vi "PreviousMonth.vi"(8 "error in (no error)":errorcluster, 11 "Calendar in":refnum<class "Calendar.lvclass">) -> (0 "error out":errorcluster, 3 "Calendar (dup)":refnum<class "Calendar.lvclass">)   [LabVIEW 2015, in "Calendar.lvclass"]
uses:
  Calendar.lvclass
  Calendar.lvclass/Calendar.ctl
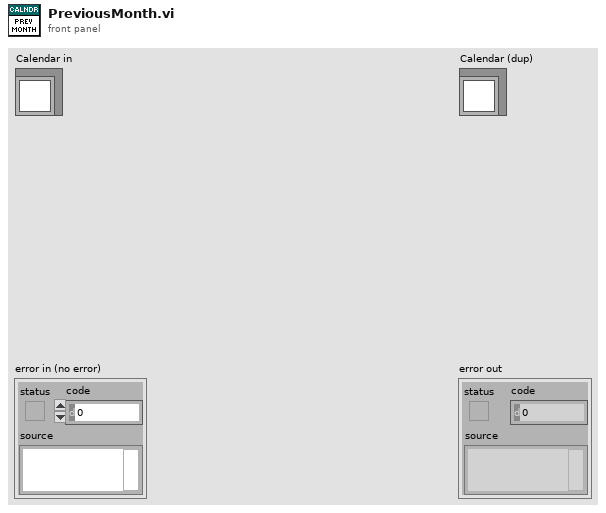
[diagram p1: front panel]
types:
  T1 = typedef "Calendar.lvclass/State Data.ctl" = cluster{"Current Date":timestamp, "First Day of Week":T2, "Color":cluster{"Selector Background":u32, "Selector Text":u32, "Days of Week Background":u32, "Days of Week Text":u32, "Calendar Background":u32, "Calendar Text":u32, "Calendar Selection Background":u32, "Calendar Selection Text":u32}, "Visible":cluster{"Today Selector Visible":bool, "Month-Year Selector Visible":bool}}
  T2 = typedef "Calendar.lvclass/DaysOfWeek.ctl" = enum16{"Sunday", "Monday", "Tuesday", "Wednesday", "Thursday", "Friday", "Saturday"}
  T3 = typedef "LVDateTimeRec.ctl" = cluster{"fractional second":dbl, "second":i32, "minute":i32, "hour":i32, "day of month":i32, "month":i32, "year":i32, "day of week":i32, "day of year":i32, "DST":i32}
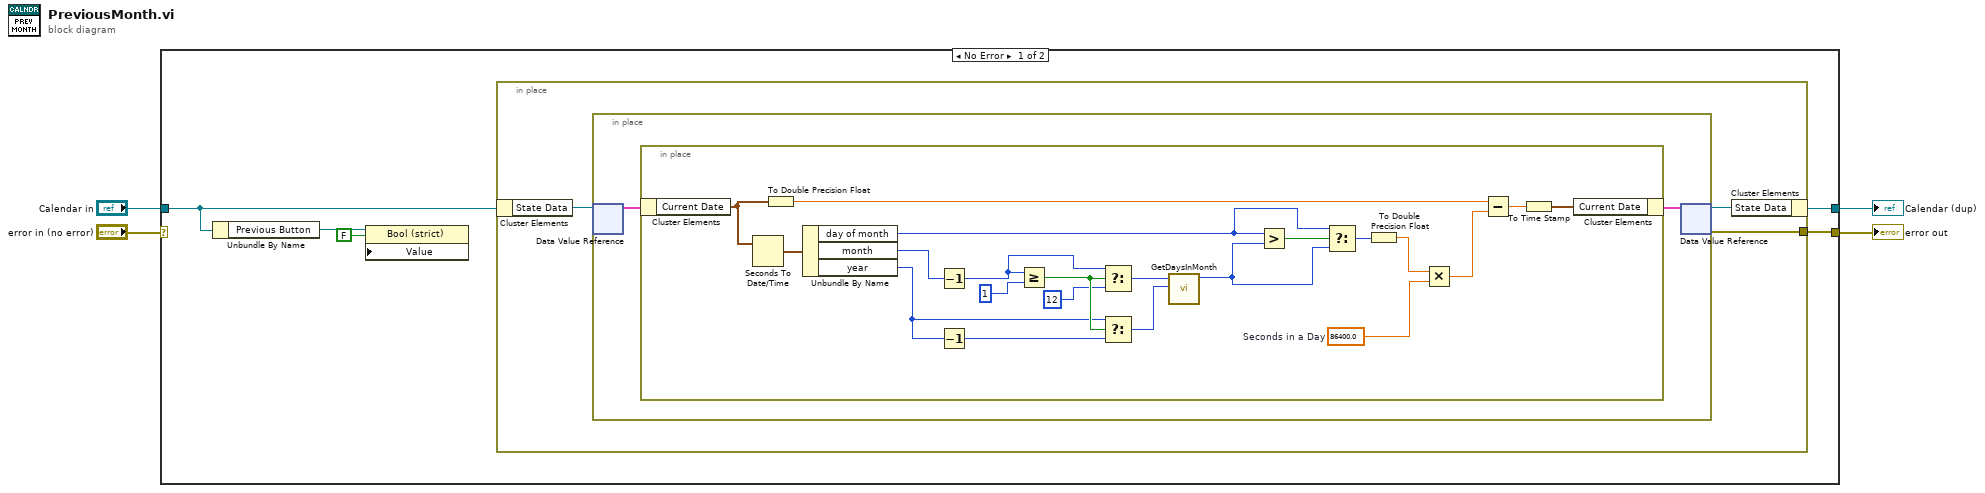
[diagram p0: block diagram]
diagram:
  n1 = case shown="No Error" "error in (no error)" {
    selector: "error in (no error)" -> [_ w37]
    tunnel: [w8 w37] -> w3
    tunnel: [w9 w36] -> w1
    tunnel: "Calendar in" -> [w7 w36]
    frame No Error {
      n2 = Unbundle By Name(w7) -> ("Previous Button"=w6:refnum<vi>)
      n3 = property class="Bool (strict)"(reference=w6, "Value"=FALSE) -> ()  [unwired: 1 in, 2 out]
      n4 = in-place {
        in-place-border: [w10] -> w8
        n5 = in-place-cluster #1(w7) -> ("State Data"=w12:refnum<data-value>)
        n6 = in-place {
          n7 = in-place-dvr #2(w12) -> (w14:T1)  [unwired: 1 out]
          n8 = in-place {
            w18 = 86400.0  # Seconds in a Day
            n9 = in-place-cluster #3(w14) -> ("Current Date"=w28:timestamp)
            n10 = Seconds To Date/Time(time stamp (now)=w28) -> (date time rec=w35:T3)  [unwired: 1 in]
            n11 = To Double Precision Float(number=w28) -> (double precision float=w27:dbl)
            n12 = Unbundle By Name(w35) -> ("day of month"=w15:i32, "month"=w24:i32, "year"=w22:i32)
            n13 = Decrement(x=w24) -> (x-1=w23:i32)
            n14 = Decrement(x=w22) -> (x-1=w34:i32)
            n15 = Greater Or Equal?(x=w23, y=1) -> (x >= y?=w33:bool)
            n16 = Select(t=w23, s=w33, f=12) -> (s? t:f=w30:i32)
            n17 = Select(t=w22, s=w33, f=w34) -> (s? t:f=w29:i32)
            n18 = call "GetDaysInMonth.vi"("Year"=w29, "Month"=w30) -> ("Number of Days in Month"=w16:i32)  [unwired: 8 in, 1 out]
            n19 = Greater?(x=w15, y=w16) -> (0:w19:bool)
            n20 = Select(t=w15, s=w19, f=w16) -> (s? t:f=w20:i32)
            n21 = To Double Precision Float(number=w20) -> (double precision float=w21:dbl)
            n22 = Multiply(x=w21, y=w18) -> (x*y=w17:dbl)
            n23 = Subtract(x=w27, y=w17) -> (x-y=w26:dbl)
            n24 = To Time Stamp(1:w26) -> (0:w25:timestamp)
            n25 = in-place-cluster #3("Current Date"=w25) -> (w13:T1)
          }
          n26 = in-place-dvr #2(w13) -> (w11:refnum<data-value>, w10:errorcluster)
        }
        n27 = in-place-cluster #1("State Data"=w11) -> (w9:refnum<class "Calendar.lvclass">)
      }
    }
    frame Error {
    }
  }
  "error out" <- w3
  "Calendar (dup)" <- w1
